vi "Append ID.vi"(9 "appended number (-1: none)":i32=-1, 10 "name":string, 11 "initial id string (\"\")":string) -> (3 "appended id string":string)   [LabVIEW 2020, in "DSF Core.lvlib" / "Configuration Session.lvclass"]
uses:
  Configuration Session.lvclass
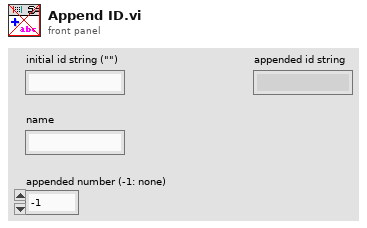
[diagram p1: front panel]
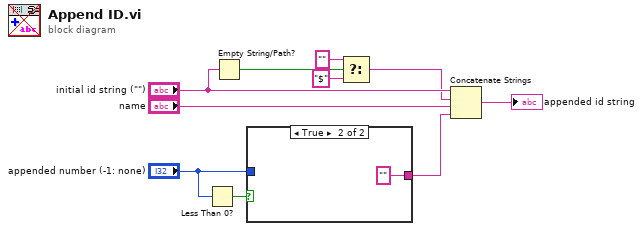
[diagram p0: block diagram]
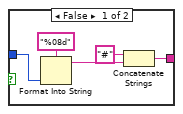
[diagram p2: hidden frame]
diagram:
  n1 = Less Than 0?(x="appended number (-1: none)") -> (x < 0?=w8:bool)
  n2 = Empty String/Path?(string/path="initial id string (\"\")") -> (empty?=w4:bool)
  n3 = case shown="True" w8 {
    tunnel: "appended number (-1: none)" -> [w13 _]
    tunnel: [w15 ""] -> w7
    frame False {
      n4 = Format Into String(format string="%08d", w13) -> (resulting string=w12:string)  [unwired: 2 in, 1 out]
      n5 = Concatenate Strings("#" ("string"), w12) -> (w15:string)
    }
    frame True {
    }
  }
  n6 = Select(t="" ("string"), s=w4, f="$") -> (s? t:f=w1:string)
  n7 = Concatenate Strings("initial id string (\"\")", w1, "name", w7) -> (→"appended id string":string)
